vi "Remove Deadband.vi"(10 "Limit":dbl, 11 "Input":dbl) -> (3 "Output":dbl)   [LabVIEW 2015]
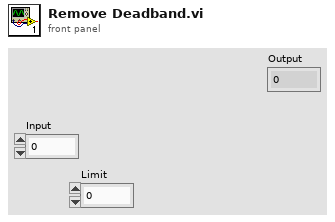
[diagram p1: front panel]
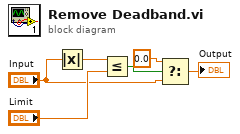
[diagram p0: block diagram]
diagram:
  n1 = Absolute Value(x="Input") -> (abs(x)=w1:dbl)
  n2 = Less Or Equal?(x=w1, y="Limit") -> (x <= y?=w6:bool)
  n3 = Select(t=0.0, s=w6, f="Input") -> (s? t:f=→"Output":dbl)
